vi "2283_driveTrain.vi"(0 "y":dbl(knob) scale=-5310.0..5310.0, 2 "x":dbl(knob) scale=-5310.0..5310.0, 3 "g":dbl(knob) scale=-5310.0..5310.0, 5 "p":dbl(knob) scale=0.0..1.0, 6 "Boton 1":bool, 8 "Boton 2":bool, 9 "angulo":dbl format="%#_13g", 10 "Boton 3":bool, 11 "angle rate":dbl format="%#_13g", 12 "Modificador":bool) -> (14 "i1":dbl(slide) scale=-1.0..1.0, 16 "d1":dbl(slide) scale=-1.0..1.0, 17 "i2":dbl(slide) scale=-1.0..1.0, 19 "d2":dbl(slide) scale=-1.0..1.0)   [LabVIEW 2014]
uses:
  <vilib>/Rock Robotics/WPI/DriverStation/WPI_DriverStationRobotMode2.ctl
  2283_Outputs autonomo.vi
  Robot Global Data.vi
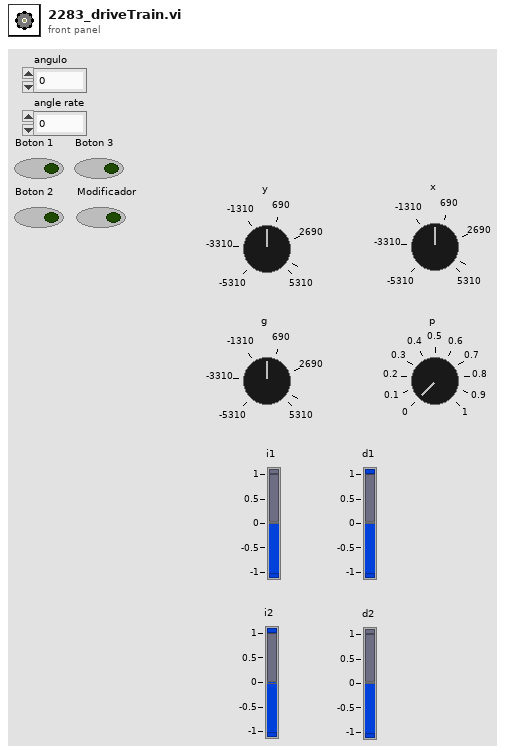
[diagram p1: front panel]
types:
  T1 = typedef "WPI_DriverStationRobotMode2.ctl" = enum16{"Autonomous Disabled", "Autonomous Enabled", "Teleop Disabled", "Teleop Enabled", "Disconnected", "Finish", "Test Disabled", "Test Enabled", "Emergency Stopped"}
  T2 = cluster{"Agarrar caja":bool, "Rotate":dbl, "Dejar caja":bool, "Activar moonwalk":bool, "Alejarse de la caja":bool, "PID LIdar":bool, "Aproach caja":bool, "Comer":bool, "Levante el bote":bool}
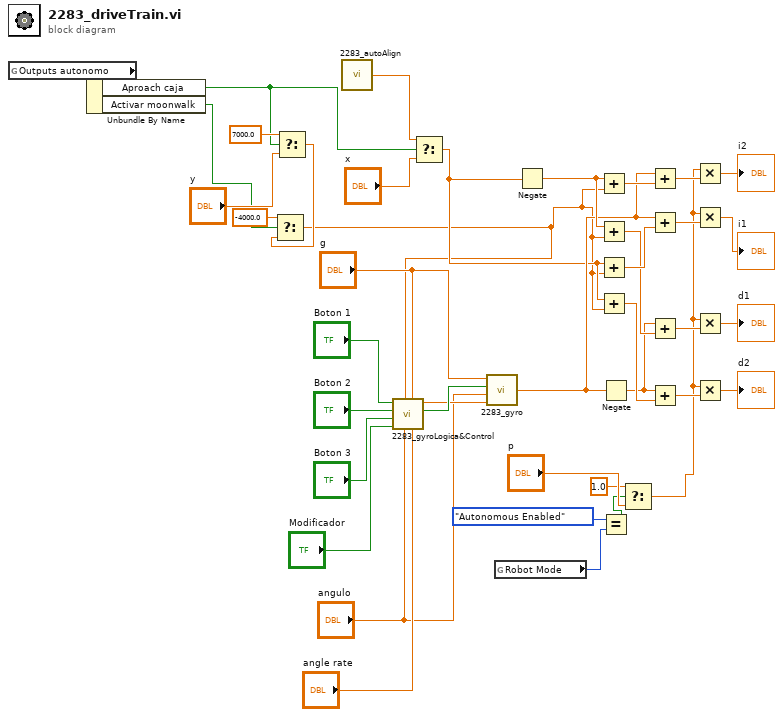
[diagram p0: block diagram]
diagram:
  n1 = global read "2283_Outputs autonomo.vi" "Outputs autonomo"() -> (w14:T2)
  n2 = Unbundle By Name(w14) -> ("Aproach caja"=w7:bool, "Activar moonwalk"=w11:bool)
  n3 = Select(t=7000.0, s=w7, f="y") -> (s? t:f=w9:dbl)
  n4 = Select(t=-4000.0, s=w11, f=w9) -> (s? t:f=w8:dbl)
  n5 = call "2283_autoAlign.vi"() -> ("output"=w15:dbl)  [unwired: 1 in]
  n6 = call "2283_gyroLogica&Control.vi"("angle rate"="angle rate", "g input"="g", "angulo"="angulo", "y input"=w8, "Modificador"="Modificador", "Boton 3"="Boton 3", "Boton 2"="Boton 2", "Boton 1"="Boton 1") -> ("g boolean"=w26:bool, "angulo deseado"=w20:dbl)  [unwired: 2 in]
  n7 = Select(t=w15, s=w7, f="x") -> (s? t:f=w16:dbl)
  n8 = call "2283_gyro.vi"("g input"="g", "g boolean"=w26, "angulo"="angulo", "angulo deseado"=w20) -> ("g output"=w27:dbl)  [unwired: 1 in]
  n9 = global read "Robot Global Data.vi" "Robot Mode"() -> (w5:T1)
  n10 = Negate(x=w16) -> (-x=w37:dbl)
  n11 = Add(x=w37, y=w8) -> (x+y=w39:dbl)
  n12 = Add(x=w37, y=w8) -> (x+y=w40:dbl)
  n13 = Add(x=w16, y=w8) -> (x+y=w41:dbl)
  n14 = Add(x=w16, y=w8) -> (x+y=w38:dbl)
  n15 = Negate(x=w27) -> (-x=w36:dbl)
  n16 = Equal?(x=WPI_DriverStationRobotMode2."Autonomous Enabled" ("Robot Mode"), y=w5) -> (x = y?=w2:bool)
  n17 = Select(t=1.0, s=w2, f="p") -> (s? t:f=w4:dbl)
  n18 = Add(x=w27, y=w39) -> (x+y=w34:dbl)
  n19 = Add(x=w27, y=w41) -> (x+y=w32:dbl)
  n20 = Add(x=w36, y=w40) -> (x+y=w33:dbl)
  n21 = Add(x=w36, y=w38) -> (x+y=w35:dbl)
  n22 = Multiply(x=w4, y=w34) -> (x*y=→"i2":dbl)
  n23 = Multiply(x=w4, y=w32) -> (x*y=→"i1":dbl)
  n24 = Multiply(x=w4, y=w33) -> (x*y=→"d1":dbl)
  n25 = Multiply(x=w4, y=w35) -> (x*y=→"d2":dbl)
